vi "TestDemo.vi"() -> ()   [LabVIEW 2018]
uses:
  Properties/Set Correct Color.vi
  Properties/Set Error Color.vi
  Properties/Set Format.vi
  SpecificString.lvclass
panel:
  in  "String":string
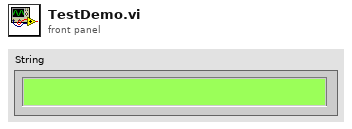
[diagram p1: front panel]
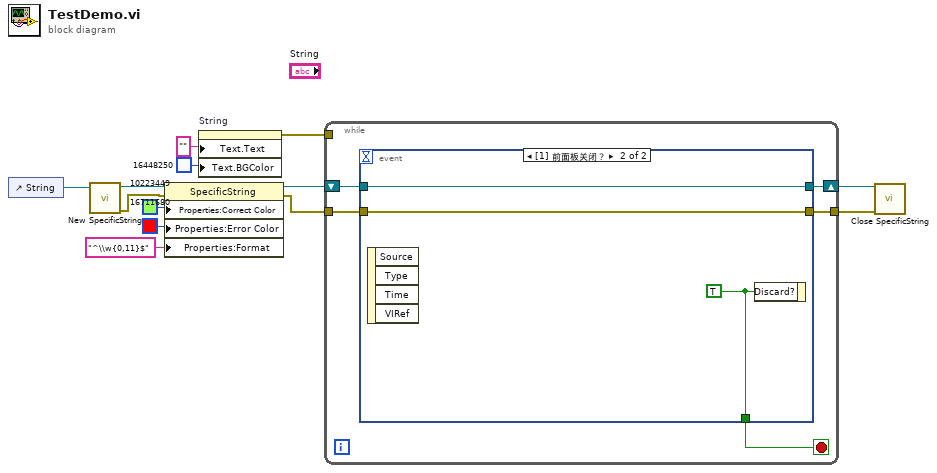
[diagram p0: block diagram]
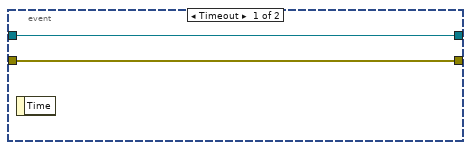
[diagram p2: hidden frame]
diagram:
  n1 = control-ref of="String"() -> (w13:refnum<vi>)
  n2 = call "New SpecificString.vi"("Reference"=w13) -> ("error out"=w4:errorcluster, "SpecificString out"=w12:refnum<class "SpecificString.lvclass">)  [unwired: 9 in]
  n3 = property class="SpecificString"(reference=w12, error in=w4, "Properties:Correct Color"=u32 10223449 ("Correct Color"), "Properties:Error Color"=u32 16711680 ("Error Color"), "Properties:Format"="^\\w{0,11}$" ("Format")) -> (reference out=w6:refnum<class "SpecificString.lvclass">, error out=w3:errorcluster)
  n4 = property on="String" class="Str"("Text.Text"="" ("文本.文本"), "Text.BGColor"=u32 16448250 ("文本.文本颜色:背景色")) -> (error out=w1:errorcluster)  [unwired: 2 in, 1 out]
  n5 = while {
    shift-right: [w17] -> w5
    shift-left: w6 -> [w18]
    tunnel: w3 -> [w16]
    tunnel: [w15] -> w2
    tunnel: w1 -> [_]
    stop <- w14 stop-if-true
    n6 = event shown="[1] 前面板关闭？" {
      selector: _ -> [_ _]
      dyn-events: _ -> [_ _]
      timeout: _ -> [_ _]
      tunnel: w18 -> [w20 w23]
      tunnel: [w20 w23] -> w17
      tunnel: w16 -> [w19 w22]
      tunnel: [w19 w22] -> w15
      tunnel: [_ w21] -> w14
      event Timeout {
        n7 = event-data() -> ()  [unwired: 1 in, 1 out]
      }
      event Panel Close? {
        w21 = TRUE ("放弃？")
        n8 = event-data() -> ()  [unwired: 1 in, 4 out]
        n9 = event-data("Discard?"=w21) -> ()  [unwired: 1 in, 1 out]
      }
    }
  }
  n10 = call "Close SpecificString.vi"("error in (no error)"=w2, "SpecificString in"=w5) -> ()  [unwired: 9 in, 1 out]
